vi "ASDOptimize.vi"(0 "TCP Network Connection Refnum":refnum<k5>, 1 "Optimize":bool, 7 "error in (no error)":errorcluster) -> (20 "Header Code":i32, 21 "Error Code":i32, 22 "VNIR Integration Time":i32, 23 "SWIR 1 Gain":i32, 24 "SWIR 2 Gain":i32, 25 "SWIR 1 Offset":i32, 26 "SWIR 2 Offset":i32, 27 "error out":errorcluster)   [LabVIEW 2010]
panel:
  # "This is a Sub-VI of ASDTCPDemo."
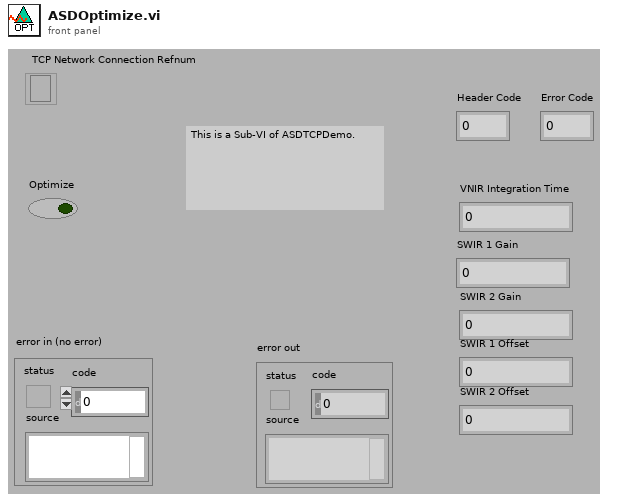
[diagram p1: front panel]
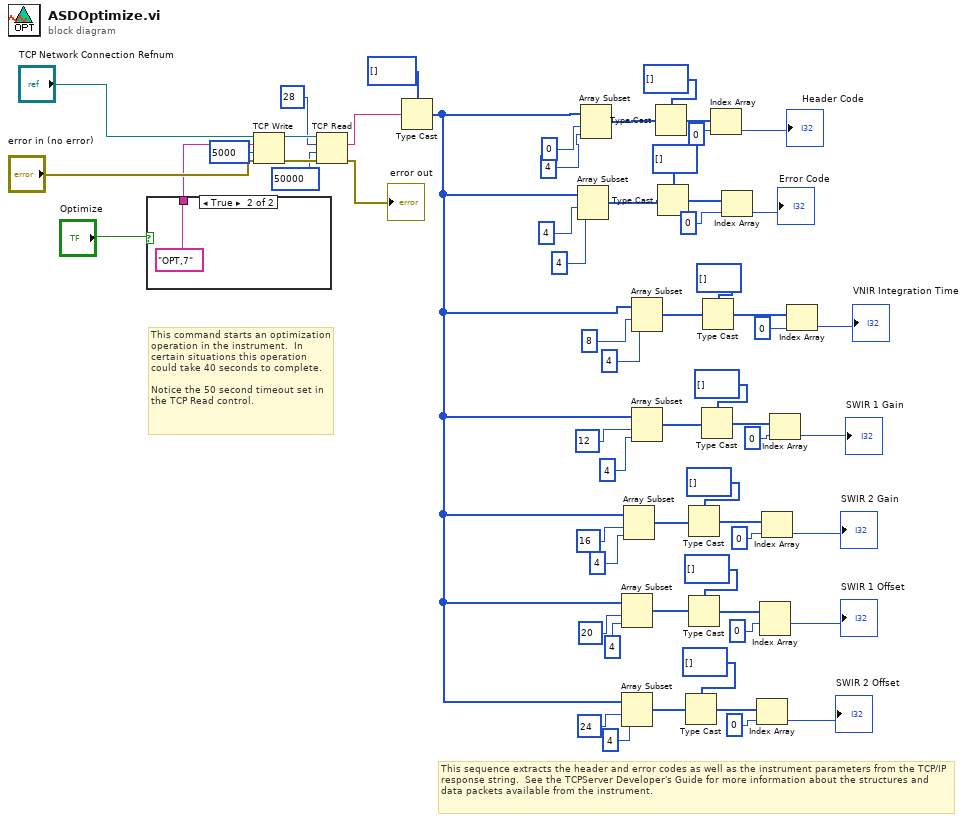
[diagram p0: block diagram]
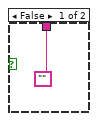
[diagram p2: hidden frame]
diagram:
  # "This sequence extracts the header and error codes as well as the instrument parameters from the TCP/IP response string.  See the TCPServer Developer's Guide for more information about the structures and data packets available from the instrument."
  # "This command starts an optimization operation in the instrument.  In certain situations this operation could take 40 seconds to complete.  \n\nNotice the 50 second timeout set in the TCP Read control."
  n1 = case shown="True" "Optimize" {
    tunnel: ["" "OPT,7"] -> w57
    frame False {
    }
    frame True {
    }
  }
  n2 = TCP Write(connection ID="TCP Network Connection Refnum", data in=w57, error in (no error)="error in (no error)", 9:5000 ("timeout ms (25000)")) -> (connection ID out=w58:refnum<k5>, error out=w59:errorcluster)  [unwired: 1 out]
  n3 = TCP Read(connection ID=w58, bytes to read=28, error in (no error)=w59, 9:50000 ("timeout ms (25000)")) -> (data out=w30:string, error out=→"error out":errorcluster)  [unwired: 1 in, 1 out]
  n4 = Type Cast(type=u8[] [], x=w30) -> (*(type *) &x=w1:u8[])
  n5 = Array Subset(array=w1, index=4, length=4 ("index")) -> (w49:u8[])
  n6 = Array Subset(array=w1, index=0 ("start index (0)"), length=4) -> (w43:u8[])
  n7 = Array Subset(array=w1, index=20, length=4 ("index")) -> (w9:u8[])
  n8 = Array Subset(array=w1, index=24, length=4 ("index")) -> (w8:u8[])
  n9 = Array Subset(array=w1, index=16, length=4 ("index")) -> (w22:u8[])
  n10 = Array Subset(array=w1, index=8, length=4 ("index")) -> (w42:u8[])
  n11 = Array Subset(array=w1, index=12, length=4 ("index")) -> (w23:u8[])
  n12 = Type Cast(type=i32[] [], x=w43) -> (*(type *) &x=w44:i32[])
  n13 = Type Cast(type=i32[] [], x=w49) -> (*(type *) &x=w48:i32[])
  n14 = Type Cast(type=i32[] [], x=w8) -> (*(type *) &x=w2:i32[])
  n15 = Type Cast(type=i32[] [], x=w22) -> (*(type *) &x=w16:i32[])
  n16 = Type Cast(type=i32[] [], x=w9) -> (*(type *) &x=w15:i32[])
  n17 = Type Cast(type=i32[] [], x=w23) -> (*(type *) &x=w29:i32[])
  n18 = Type Cast(type=i32[] [], x=w42) -> (*(type *) &x=w35:i32[])
  n19 = Index Array(array=w44, index=0) -> (element=→"Header Code":i32)
  n20 = Index Array(array=w48, index=0) -> (element=→"Error Code":i32)
  n21 = Index Array(array=w2, index=0) -> (element=→"SWIR 2 Offset":i32)
  n22 = Index Array(array=w15, index #1=0 ("index")) -> (element #1=→"SWIR 1 Offset":i32)  [unwired: 1 in, 1 out]
  n23 = Index Array(array=w16, index=0) -> (element=→"SWIR 2 Gain":i32)
  n24 = Index Array(array=w29, index=0) -> (element=→"SWIR 1 Gain":i32)
  n25 = Index Array(array=w35, index=0) -> (element=→"VNIR Integration Time":i32)
